vi "FGV SystemEinstellungenV2.vi"(6 "Aktion":T7, 8 "error in (no error)":errorcluster caption="Fehler (Eingang, kein Fehler)", 10 "Gasteiler definition":T1 {"Gasteiler Letzte Wartung" format="%<%x %.3X>T"}, 11 "AnalysatorDefinition":T3) -> (0 "error out":errorcluster caption="Fehler (Ausgang)", 2 "Gasteiler":T2 {"GasteilerDefinitionsListe"."Gasteiler Letzte Wartung" format="%<%x %.3X>T"}, 3 "Analysatoren":T5, 4 "Untertitel":T6, 5 "Index Neuer analysator":i32, 7 "Index Neuer Gasteiler":i32)   [LabVIEW 2020, in "System Einstellungen V2.lvlib"]
uses:
  System Einstellungen V2.lvlib
  Aktion FGV SystemEinstellungenV2.ctl
  AnalysatorDefinition.ctl
  Gasteiler.ctl
  <vilib>/Utility/miscctls.llb/LVComboBoxStrsAndValuesArrayTypeDef.ctl
  EPA 1065/Allgemeine VIs/Aktion Wertaenderung Gasliste.ctl
  Aktioen FGV System.ctl
  SysLog/SysLog Interface.ctl
  Allgemein/allgemeine Sub-VIs.lvlib
  SysLog/SysLog.lvlib
  EPA 1065/EPA 1065.lvlib
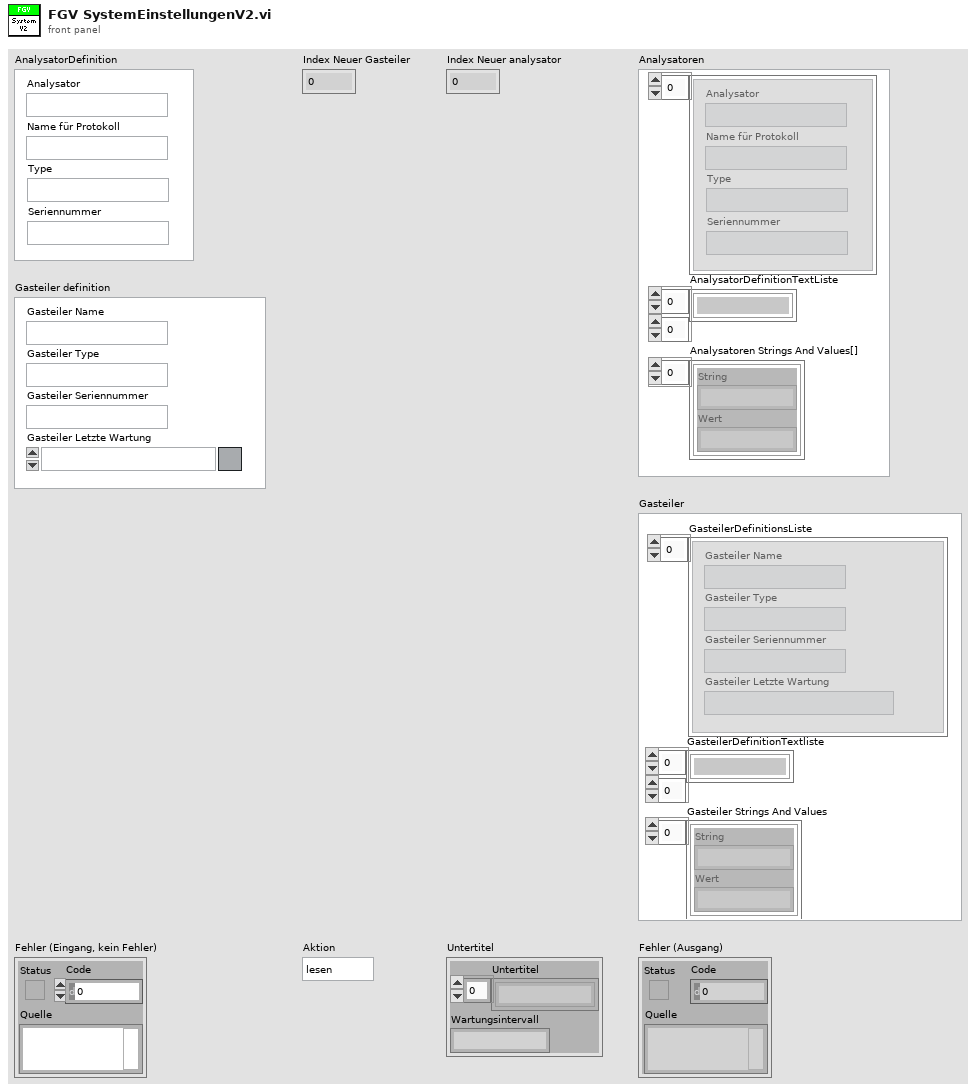
[diagram p1: front panel]
types:
  T1 = typedef "System Einstellungen V2.lvlib/Gasteiler.ctl" = cluster{"Gasteiler Name":string, "Gasteiler Type":string, "Gasteiler Seriennummer":string, "Gasteiler Letzte Wartung":timestamp}
  T2 = cluster{"GasteilerDefinitionsListe":T1[], "GasteilerDefinitionTextliste":string[][], "Gasteiler Strings And Values":cluster{"String":string, "Wert":string}[]}
  T3 = typedef "System Einstellungen V2.lvlib/AnalysatorDefinition.ctl" = cluster{"Analysator":string, "Name für Protokoll":string, "Type":string, "Seriennummer":string}
  T4 = typedef "LVComboBoxStrsAndValuesArrayTypeDef.ctl" = cluster{"String":string, "Value":string}[]
  T5 = cluster{"AnalysatorDefinitionListe":T3[], "AnalysatorDefinitionTextListe":string[][], "Analysatoren Strings And Values[]":T4}
  T6 = cluster{"Untertitel":string[], "Wartungsintervall":string}
  T7 = typedef "System Einstellungen V2.lvlib/Aktion FGV SystemEinstellungenV2.ctl" = enum16{"lesen", "Analysatoren schreiben", "Analysator ändern", "Analysatoren löschen", "laden", "speichern", "Untertitel", "Analysatoren", "Neue Analysatoren", "Gasteiler schreiben", "Gasteiler ändern", "Gasteiler löschen", "Gasteiler", "Gasteiler exportieren", "Gasteiler importieren"}
  T8 = enum16{"open", "replace", "create", "open or create", "replace or create", "replace or create with confirmation"}
  T9 = typedef "EPA 1065.lvlib/Aktion Wertaenderung Gasliste.ctl" = enum16{"Init", "lesen", "Gasliste geändert", "ARN inaktiv", "LEAK inaktiv", "Interference 366 inaktiv", "T90 inaktiv", "Interference 375 inaktiv", "Chiller inaktiv", "FID O2 inaktiv", "FID Opti inaktiv", "Drift inaktiv", "Pre Test inaktiv", "LinV2 inaktiv"}
  T10 = typedef "System Einstellungen V2.lvlib/Aktioen FGV System.ctl" = enum16{"lesen", "laden", "speichern", "Optionen schreiben", "Zeitstempel", "Reset BMP", "Reset SQP", "Wartung", "Werkseinstellung"}
  T11 = typedef "SysLog.lvlib/SysLog Interface.ctl" = cluster{"FehlermeldungsCode":i32, "ErfolgsmeldungsCode":i32, "ParameterListenString":string, "Anzeige":bool, "SysLogIcon":enum16{"OK", "Warnung", "Fehler"}, "intern":bool}
  T12 = cluster{"Gasteiler Name":string, "Gasteiler Name":string}
  T13 = cluster{"Analysator":string, "Analysator":string}[]
  T14 = typedef "System Einstellungen V2.lvlib/Optionen.ctl" = cluster{"Störmeldep.":bool, "Betriebszustände":bool, "AK in ppm":bool, "log Cal-Gas":bool, "log 0-Gas":bool, "Durchflusssensor 0-5V":bool, "PNS?":bool, "Mit N2 spülen":bool, "TRE08":bool, "Amium 10-Fach":bool, "Verticale Scrollbar aktiv":bool, "Loggingtakt":bool, "AK Rezeptwechsel gleich wie MKS":bool, "NG ECO":bool}
  T15 = cluster{"Cluster Array (Ausgang)":T1[], "Gasteiler definition":string[][], cluster{"Gasteiler Name":string, "Gasteiler Name":string}[]}
  T16 = cluster{"AnalysatorDefinition Array out":T3[], "Analysator String Array out":string[][], "Analysatoren Strings And Values[]":cluster{"Analysator":string, "Analysator":string}[]}
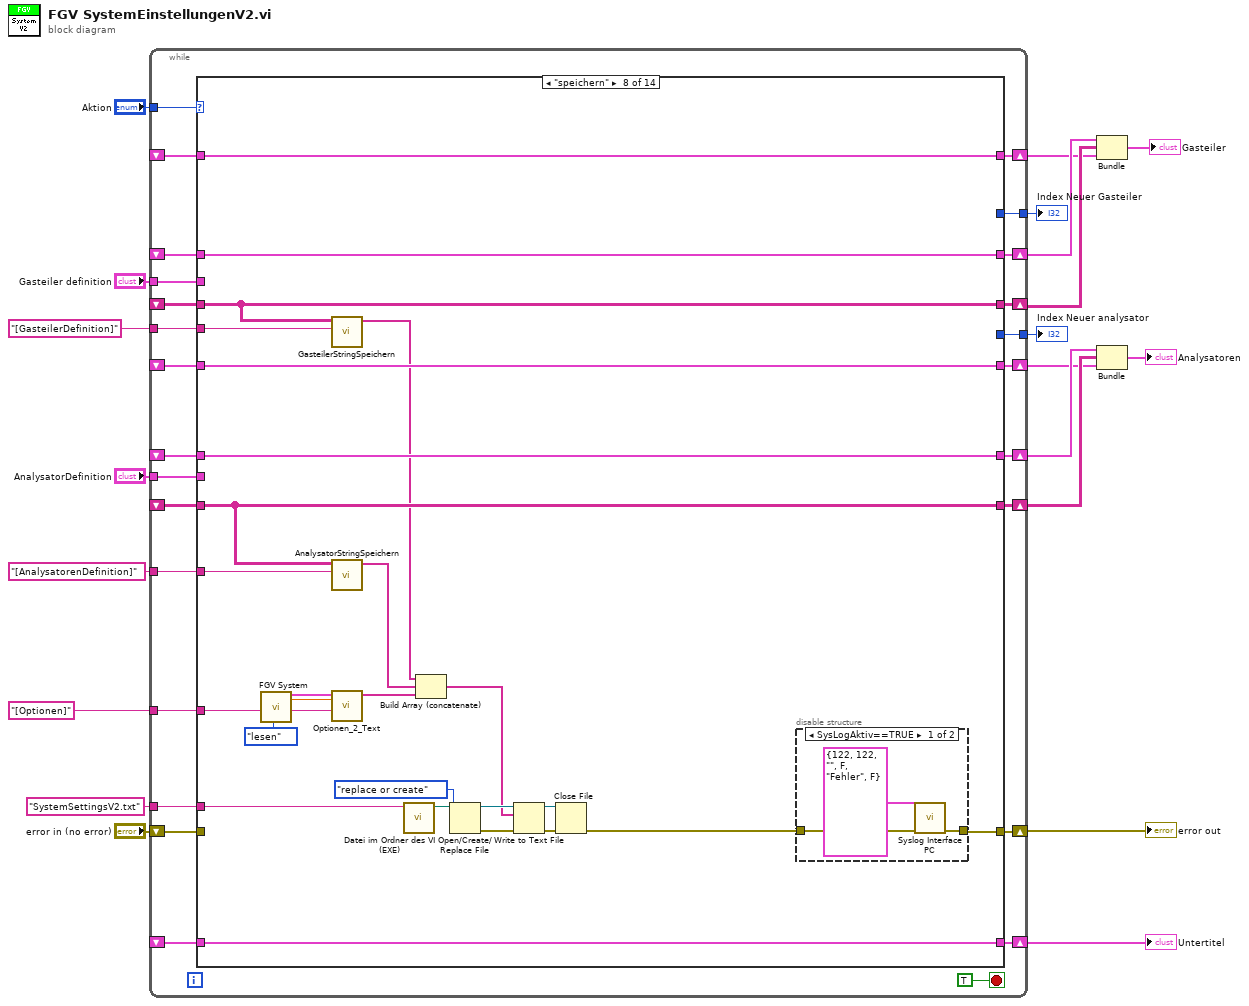
[diagram p0: block diagram]
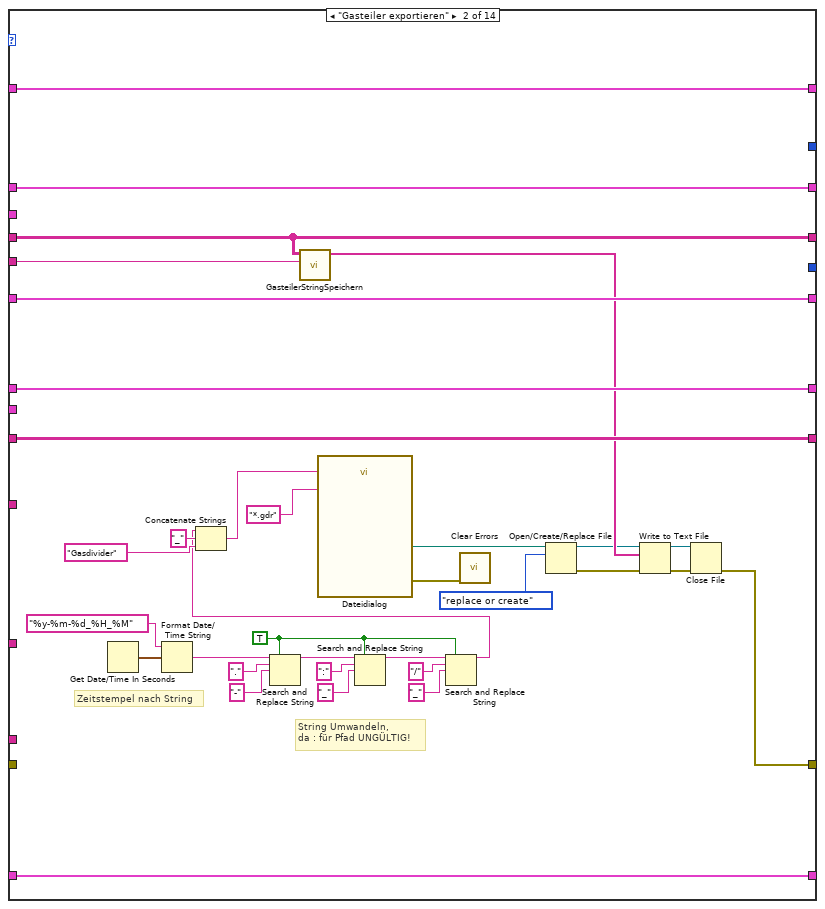
[diagram p3: hidden frame]
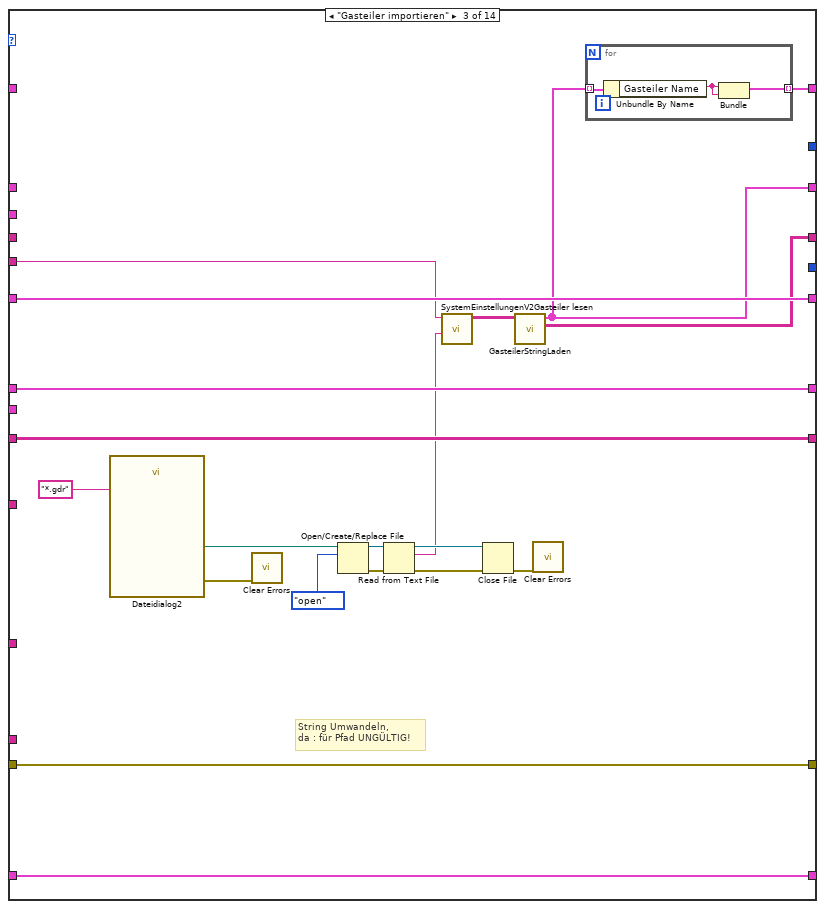
[diagram p4: hidden frame]
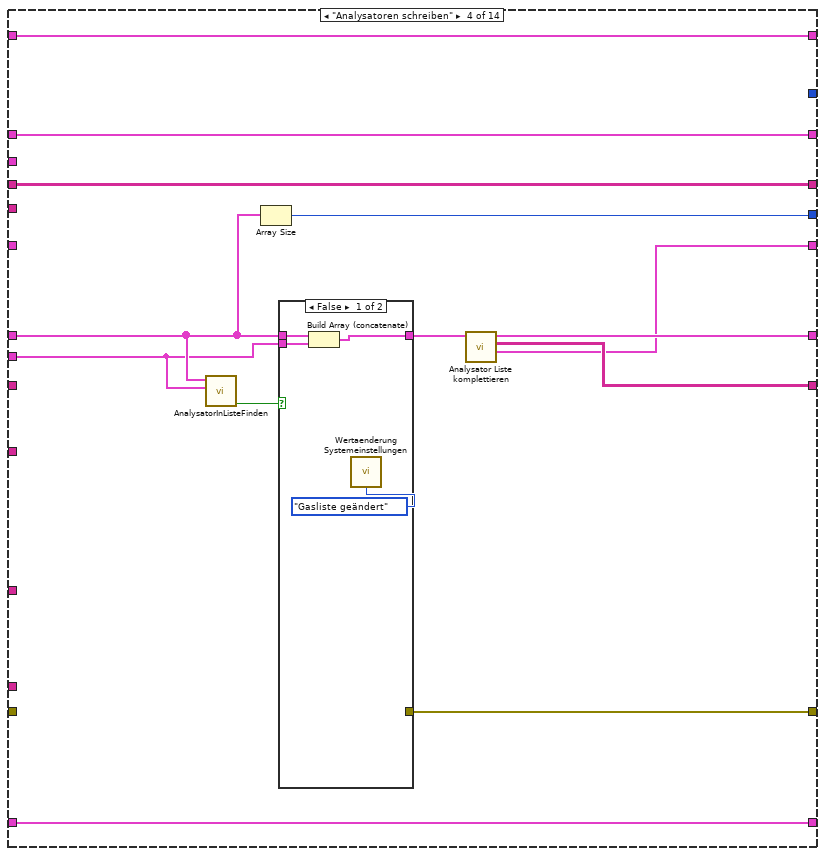
[diagram p5: hidden frame]
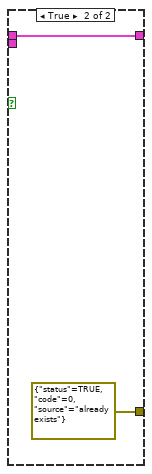
[diagram p6: hidden frame]
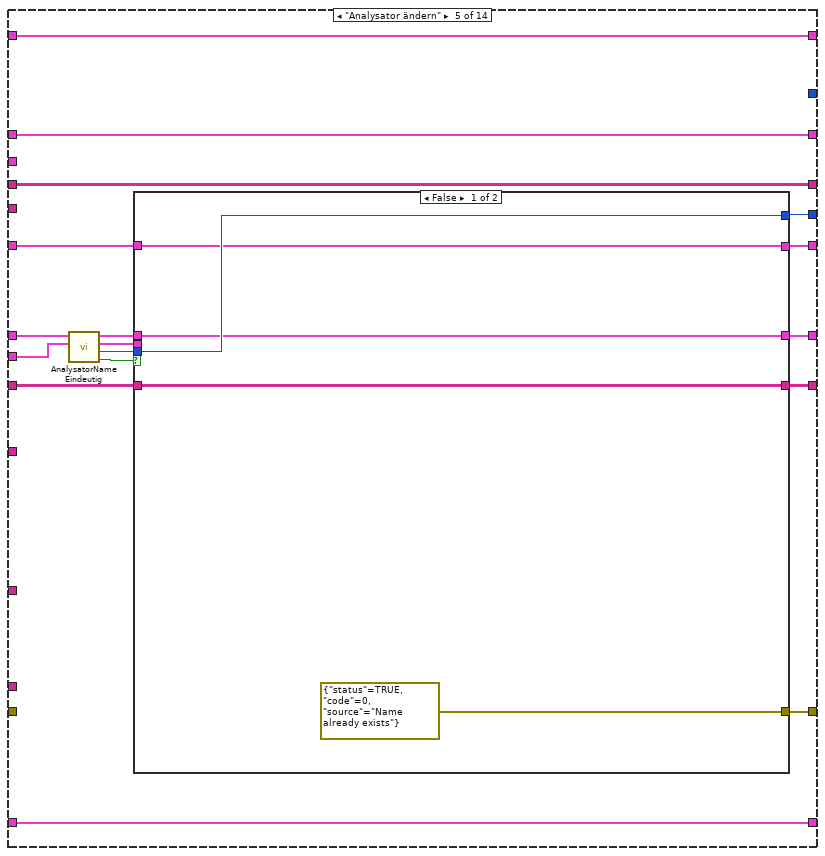
[diagram p7: hidden frame]
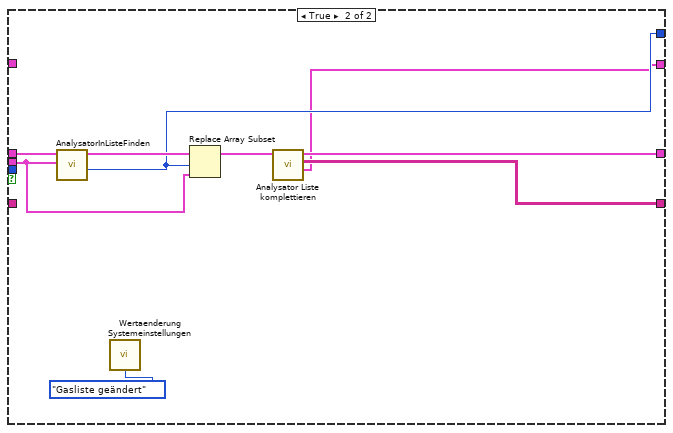
[diagram p8: hidden frame]
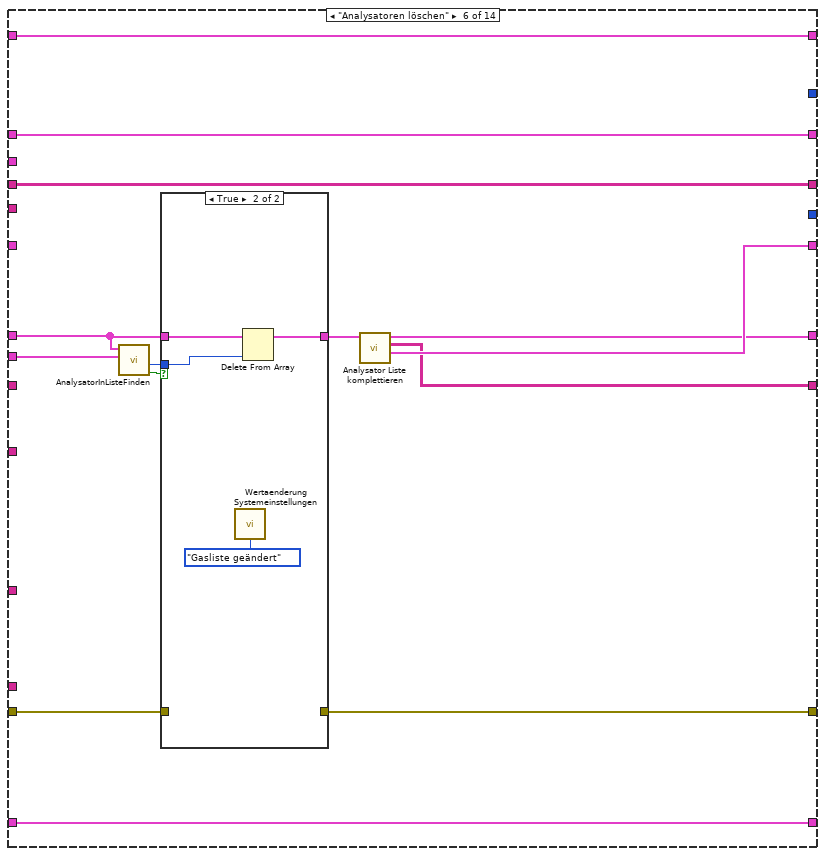
[diagram p9: hidden frame]
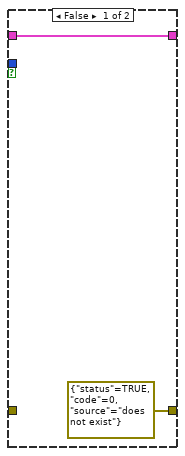
[diagram p10: hidden frame]
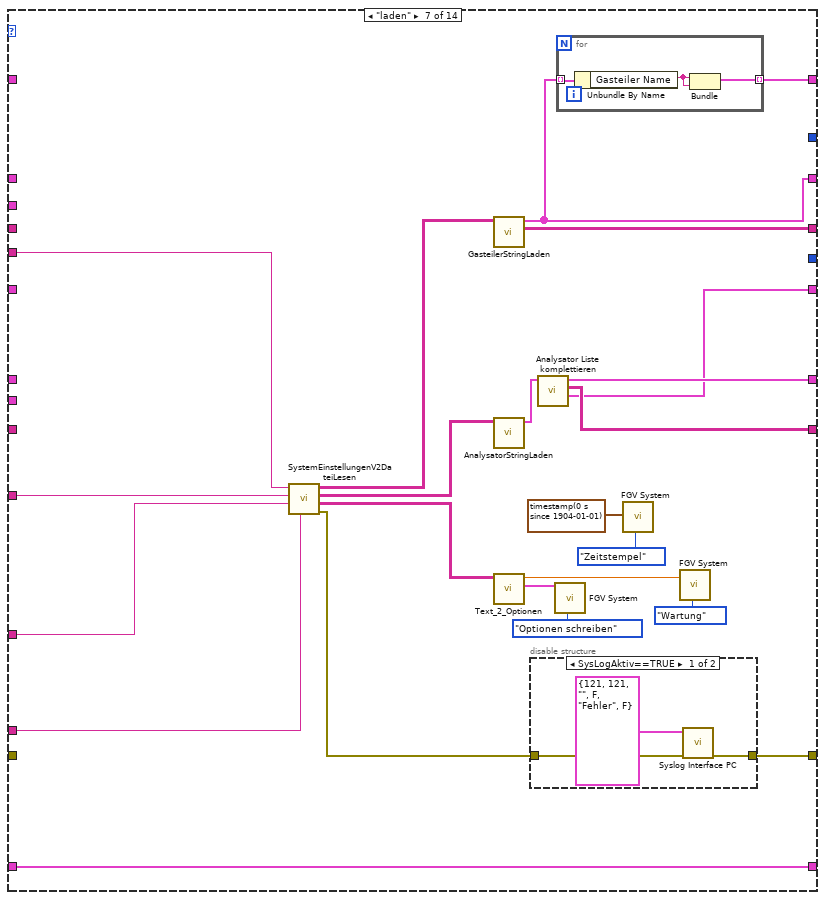
[diagram p11: hidden frame]
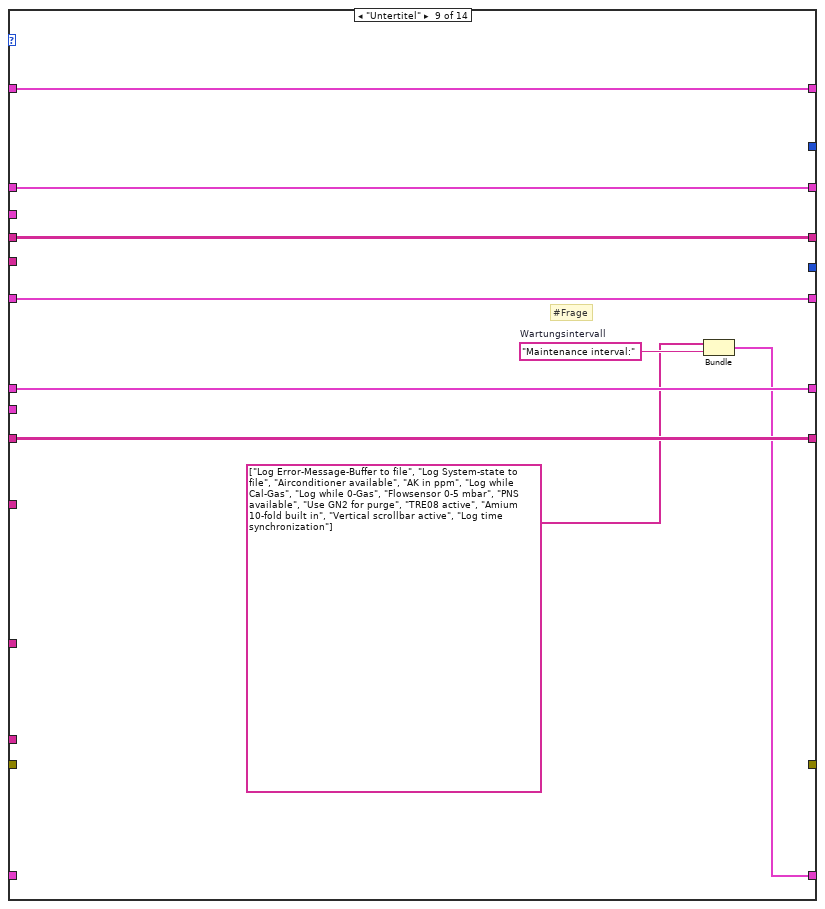
[diagram p14: hidden frame]
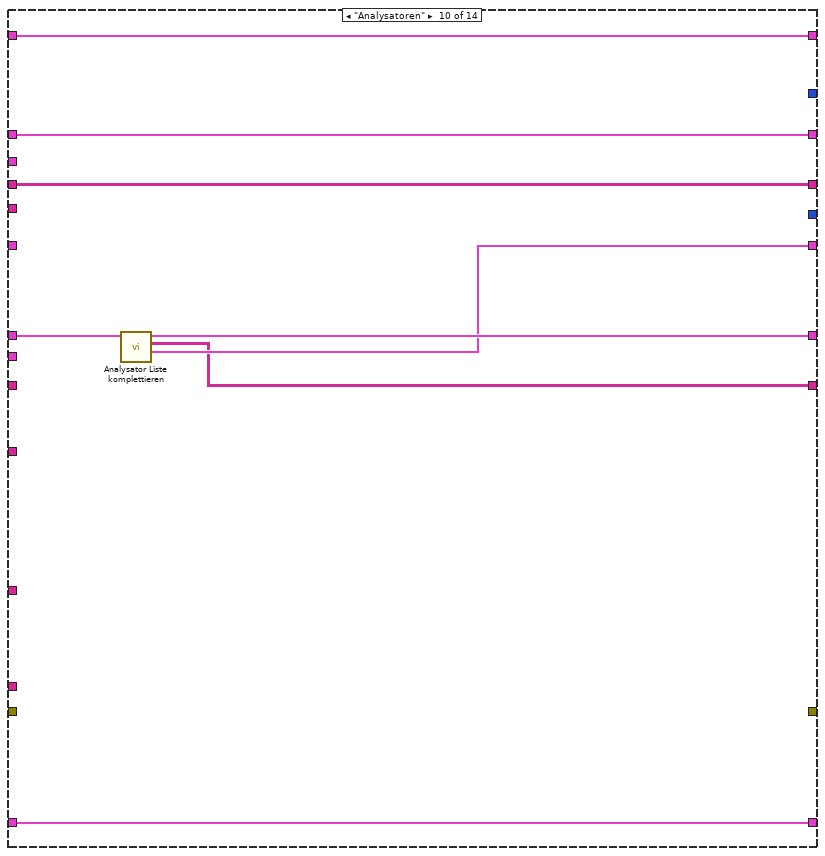
[diagram p15: hidden frame]
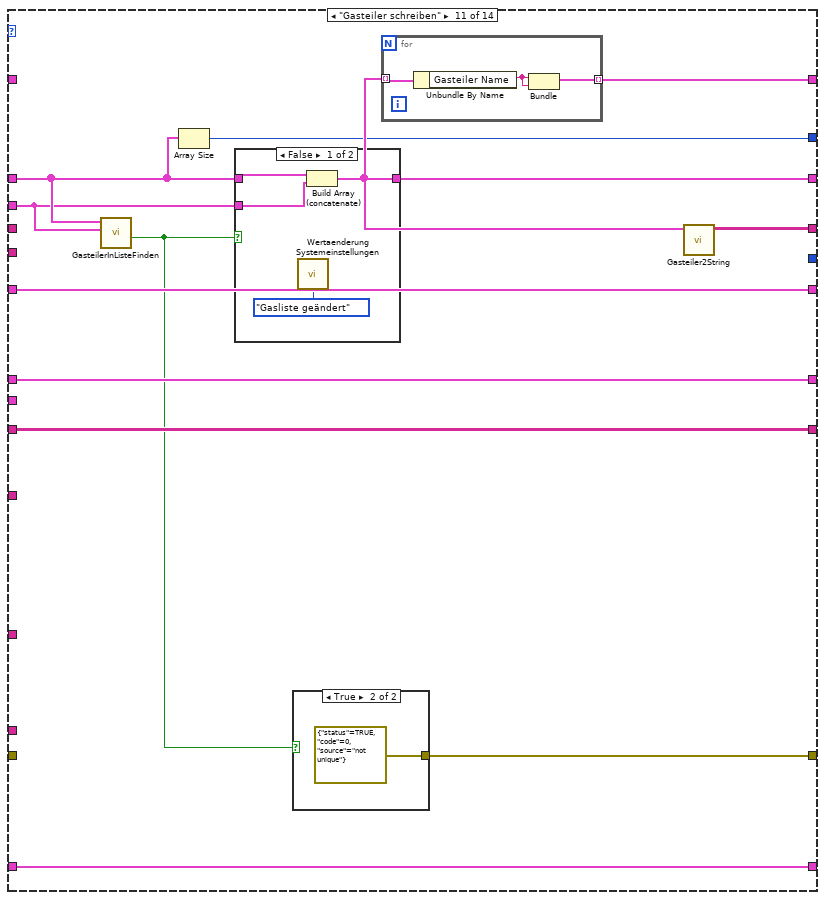
[diagram p16: hidden frame]
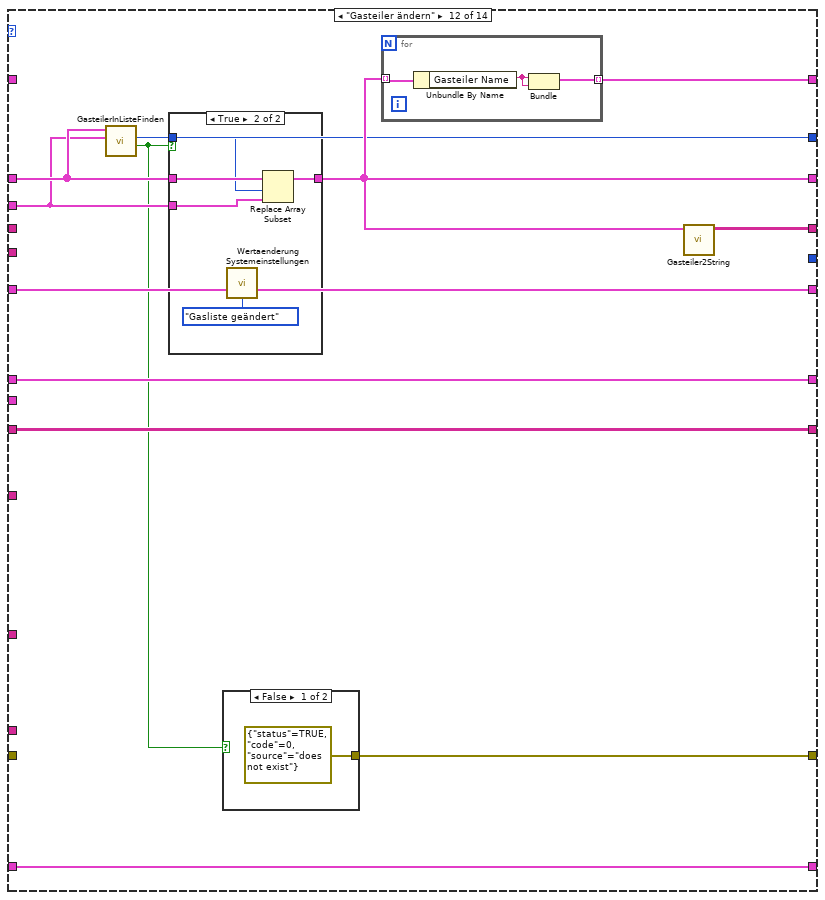
[diagram p19: hidden frame]
diagram:
  n1 = while {
    tunnel: "Aktion" -> [w45]
    shift-right: [w44] -> w12
    shift-left: _ -> [w43]
    shift-right: [w42] -> w11
    shift-left: _ -> [w41]
    shift-right: [w39] -> w18
    shift-left: "error in (no error)" -> [w40]
    tunnel: "SystemSettingsV2.txt" ("Dateiname") -> [w38]
    tunnel: "[AnalysatorenDefinition]" -> [w37]
    tunnel: "AnalysatorDefinition" -> [w36]
    tunnel: "[Optionen]" -> [w35]
    shift-right: [w34] -> w13
    shift-left: _ -> [w33]
    shift-right: [w32] -> w10
    shift-left: _ -> [w31]
    tunnel: "Gasteiler definition" -> [w30]
    shift-right: [w29] -> w7
    shift-left: _ -> [w28]
    shift-right: [w27] -> w6
    shift-left: _ -> [w26]
    shift-right: [w25] -> w5
    shift-left: _ -> [w24]
    tunnel: "[GasteilerDefinition]" -> [w23]
    tunnel: [w22] -> w2
    tunnel: [w21] -> w1
    stop <- TRUE stop-if-true
    n2 = case shown="\"speichern\"" w45 {
      tunnel: [w54 w88 w108 w114 w137 w163 w184 w237 w250 w253 w270 w291 w314 w330] -> w44
      tunnel: w43 -> [w54 w88 w108 w119 w142 w173 _ w237 w250 w254 w270 w291 w314 w330]
      tunnel: [w53 w87 w107 w113 w135 w162 w183 w229 w249 w251 w269 w290 w313 w329] -> w42
      tunnel: w41 -> [w53 w87 w107 _ w131 _ _ w229 w249 _ w269 w290 w313 w329]
      tunnel: w40 -> [w52 _ w106 _ _ w175 _ _ _ _ _ _ w306 _]
      tunnel: [w52 w55 w106 w116 w146 w174 w186 w214 _ _ w259 w287 w307 _] -> w39
      tunnel: w38 -> [_ _ _ _ _ _ w204 w230 _ _ _ _ _ _]
      tunnel: w37 -> [_ _ _ _ _ _ w190 w212 _ _ _ _ _ _]
      tunnel: w36 -> [_ _ _ w118 w141 w172 _ _ _ _ _ _ _ _]
      tunnel: w35 -> [_ _ _ _ _ _ w189 w222 _ _ _ _ _ _]
      tunnel: [w51 w86 w105 w124 w147 w171 w196 w221 w248 w258 w268 w289 w312 w328] -> w34
      tunnel: w33 -> [w51 w86 w105 w124 w147 w171 w196 w221 _ w258 w268 w289 w312 w328]
      tunnel: [w50 w85 w104 w112 w134 w165 w182 w220 w246 w252 w267 w288 w311 w327] -> w32
      tunnel: w31 -> [w50 w85 w104 _ w132 _ _ w220 w246 _ w267 w288 w311 w327]
      tunnel: w30 -> [_ _ _ _ _ _ _ _ _ _ w262 w282 w308 _]
      tunnel: [w49 w63 w92 w123 w145 w170 w192 w219 w245 w257 w266 w286 w302 w325] -> w29
      tunnel: w28 -> [w49 w63 _ w123 w145 w170 _ w219 w245 w257 w263 w283 w305 w325]
      tunnel: [w48 w62 w91 w122 w144 w169 w193 w217 w244 w256 w265 w285 w303 w326] -> w27
      tunnel: w26 -> [w48 w62 _ w122 w144 w169 _ w217 w244 w256 _ _ _ w326]
      tunnel: [w47 w64 w93 w121 w143 w168 w191 w218 w243 w255 w264 w284 w304 w324] -> w25
      tunnel: w24 -> [w47 w64 _ w121 w143 w168 _ w218 w243 w255 _ _ _ _]
      tunnel: w23 -> [_ w61 w90 _ _ _ w195 w213 _ _ _ _ _ _]
      tunnel: [_ _ _ _ _ _ _ _ _ _ w261 w281 _ _] -> w22
      tunnel: [_ _ _ w120 w136 _ _ _ _ _ _ _ _ _] -> w21
      frame "lesen", Default {
      }
      frame "Gasteiler exportieren" {
        w72 = TRUE ("Alle ersetzen? (F)")
        # "String Umwandeln, \nda : für Pfad UNGÜLTIG!"
        # "Zeitstempel nach String"
        n3 = Get Date/Time In Seconds() -> (seconds since 1Jan1904=w82:timestamp)
        n4 = Format Date/Time String(time format string (%c)="%y-%m-%d_%H_%M" ("Zeitformatierungs-String (%c)"), seconds (now)=w82) -> (date/time string=w81:string)  [unwired: 1 in]
        n5 = Search and Replace String(replace all?=w72, input string=w81, search string="." ("Such-String"), replace string="-" ("String ersetzen(\"\")")) -> (result string=w78:string)  [unwired: 4 in, 3 out]
        n6 = call "GasteilerStringSpeichern.vi"("Abschnitt"=w61, "GasteilerDefinition"=w62) -> ("Gasdivider Text to save"=w60:string[])  [unwired: 9 in]
        n7 = Search and Replace String(replace all?=w72, input string=w78, search string=":" ("Such-String"), replace string="_" ("String ersetzen(\"\")")) -> (result string=w73:string)  [unwired: 4 in, 3 out]
        n8 = Search and Replace String(replace all?=w72, input string=w73, search string="/" ("Such-String"), replace string="_" ("String ersetzen(\"\")")) -> (result string=w68:string)  [unwired: 4 in, 3 out]
        n9 = Concatenate Strings(w68, "_" ("String"), "Gasdivider" ("default name")) -> (w67:string)
        n10 = call "Dateidialog"("default name"=w67, "pattern (all files)"="*.gdr") -> ("selected path"=w66:path, "error out"=w83:errorcluster)  [unwired: 10 in, 2 out]
        n11 = call <vilib>:"Clear Errors.vi"("error in (no error)"=w83) -> ()  [unwired: 5 in, 2 out]
        n12 = Open/Create/Replace File(file path (use dialog)=w66, operation (0:open)=T8."replace or create" ("Operation (0:open)")) -> (refnum out=w59:refnum<file>, error out=w58:errorcluster)  [unwired: 4 in, 1 out]
        n13 = Write to Text File(file (use dialog)=w59, text=w60, error in=w58) -> (refnum out=w56:refnum<file>, error out=w57:errorcluster)  [unwired: 1 in, 1 out]
        n14 = Close File(refnum=w56, error in=w57) -> (error out=w55:errorcluster)  [unwired: 1 out]
      }
      frame "Gasteiler importieren" {
        # "String Umwandeln, \nda : für Pfad UNGÜLTIG!"
        n15 = call "Dateidialog2"("pattern (all files)"="*.gdr") -> ("selected path"=w101:path, "error out"=w102:errorcluster)  [unwired: 11 in, 2 out]
        n16 = call <vilib>:"Clear Errors.vi"("error in (no error)"=w102) -> ()  [unwired: 5 in, 2 out]
        n17 = Open/Create/Replace File(file path (use dialog)=w101, operation (0:open)=T8."open" ("Operation (0:open)")) -> (refnum out=w98:refnum<file>, error out=w97:errorcluster)  [unwired: 4 in, 1 out]
        n18 = Read from Text File(file (use dialog)=w98, error in=w97) -> (refnum out=w95:refnum<file>, text=w89:string, error out=w96:errorcluster)  [unwired: 2 in, 1 out]
        n19 = call "SystemEinstellungenV2Gasteiler lesen.vi"("Tabellen-String"=w89, "[GasteilerDefinition]"=w90) -> ("[GasteilerDefinition]"=w94:string[][])  [unwired: 8 in, 1 out]
        n20 = Close File(refnum=w95, error in=w96) -> (error out=w99:errorcluster)  [unwired: 1 out]
        n21 = call "GasteilerStringLaden.vi"("Array (Eingang)"=w94) -> ("string array"=w91:string[][], "Cluster Array (Ausgang)"=w92:T1[])  [unwired: 9 in]
        n22 = call <vilib>:"Clear Errors.vi"("error in (no error)"=w99) -> ()  [unwired: 5 in, 2 out]
        n23 = for {
          tunnel: w92 -> [w111] mode=indexing
          tunnel: [w110] -> w93 mode=indexing
          n24 = Unbundle By Name(w111) -> ("Gasteiler Name"=w109:string)
          n25 = Bundle("Gasteiler Name"=w109, "Gasteiler Name"=w109) -> (w110:T12)  [unwired: 1 in]
        }
      }
      frame "Analysatoren schreiben" {
        n26 = call "AnalysatorInListeFinden.vi"("AnalysatorDefinition"=w118, "AnalysatorListe"=w119) -> ("gefunden"=w117:bool)  [unwired: 6 in, 3 out]
        n27 = Array Size(array=w119) -> (size(s)=w120:i32)
        n28 = case shown="False" w117 {
          tunnel: [w128 w130] -> w115
          tunnel: w119 -> [w127 w130]
          tunnel: w118 -> [w126 _]
          tunnel: [_ errorcluster {"status"=TRUE, "code"=0, "source"="already exists"} ("error in (no error)")] -> w116
          frame False {
            n29 = Build Array (concatenate)(w127, w126) -> (w128:T3[])
            n30 = call "Wertaenderung Systemeinstellungen.vi"("Aktion"=Aktion_Wertaenderung_Gasliste."Gasliste geändert") -> ()  [unwired: 13 in, 2 out]
          }
          frame True {
          }
        }
        n31 = call "Analysator Liste komplettieren.vi"("AnalysatorDefinition Array in"=w115) -> ("Analysatoren Strings And Values[]"=w112:T13, "Analysator String Array out"=w113:string[][], "AnalysatorDefinition Array out"=w114:T3[])  [unwired: 8 in]
      }
      frame "Analysator ändern" {
        n32 = call "AnalysatorNameEindeutig.vi"("AnalysatorDefinition"=w141, "AnalysatorListe"=w142) -> ("unique"=w140:bool, "Index"=w133:i32, "AnalysatorDefinition out"=w139:T3, "AnalysatorListe out"=w138:T3[])  [unwired: 6 in]
        n33 = case shown="False" w140 {
          tunnel: [errorcluster {"status"=TRUE, "code"=0, "source"="Name already exists"} ("error in (no error)") _] -> w146
          tunnel: w139 -> [_ w153]
          tunnel: w138 -> [w148 w159]
          tunnel: [w148 w156] -> w137
          tunnel: [w152 w158] -> w136
          tunnel: [w149 w155] -> w135
          tunnel: [w150 w154] -> w134
          tunnel: w133 -> [w152 _]
          tunnel: w132 -> [w150 _]
          tunnel: w131 -> [w149 _]
          frame False {
          }
          frame True {
            n34 = call "AnalysatorInListeFinden.vi"("AnalysatorDefinition"=w153, "AnalysatorListe"=w159) -> ("Index"=w158:i32, "AnalysatorListe out"=w160:T3[])  [unwired: 6 in, 2 out]
            n35 = call "Wertaenderung Systemeinstellungen.vi"("Aktion"=Aktion_Wertaenderung_Gasliste."Gasliste geändert") -> ()  [unwired: 13 in, 2 out]
            n36 = Replace Array Subset(array=w160, new element=w153, index=w158) -> (w157:T3[])
            n37 = call "Analysator Liste komplettieren.vi"("AnalysatorDefinition Array in"=w157) -> ("Analysatoren Strings And Values[]"=w154:T13, "Analysator String Array out"=w155:string[][], "AnalysatorDefinition Array out"=w156:T3[])  [unwired: 8 in]
          }
        }
      }
      frame "Analysatoren löschen" {
        n38 = call "AnalysatorInListeFinden.vi"("AnalysatorDefinition"=w172, "AnalysatorListe"=w173) -> ("gefunden"=w167:bool, "Index"=w166:i32)  [unwired: 6 in, 2 out]
        n39 = case shown="True" w167 {
          tunnel: [w177 w180] -> w164
          tunnel: w173 -> [w177 w181]
          tunnel: [errorcluster {"status"=TRUE, "code"=0, "source"="does not exist"} ("error in (no error)") _] -> w174
          tunnel: w175 -> [_ _]
          tunnel: w166 -> [_ w178]
          frame False {
          }
          frame True {
            n40 = call "Wertaenderung Systemeinstellungen.vi"("Aktion"=Aktion_Wertaenderung_Gasliste."Gasliste geändert") -> ()  [unwired: 13 in, 2 out]
            n41 = Delete From Array(array=w181, index=w178) -> (array with subset deleted=w180:T3[])  [unwired: 1 in, 1 out]
          }
        }
        n42 = call "Analysator Liste komplettieren.vi"("AnalysatorDefinition Array in"=w164) -> ("Analysatoren Strings And Values[]"=w165:T13, "Analysator String Array out"=w162:string[][], "AnalysatorDefinition Array out"=w163:T3[])  [unwired: 8 in]
      }
      frame "laden" {
        n43 = call "SystemEinstellungenV2DateiLesen.vi"("Dateiname"=w204, "[Optionen]"=w189, "[AnalysatorenDefinition]"=w190, "[GasteilerDefinition]"=w195) -> ("Fehler (Ausgang)"=w203:errorcluster, "[Optionen]"=w187:string[][], "[AnalysatorenDefinition]"=w188:string[][], "[GasteilerDefinition]"=w194:string[][])  [unwired: 4 in]
        n44 = call "GasteilerStringLaden.vi"("Array (Eingang)"=w194) -> ("string array"=w193:string[][], "Cluster Array (Ausgang)"=w192:T1[])  [unwired: 9 in]
        n45 = call "AnalysatorStringLaden.vi"("Array (Eingang)"=w188) -> ("Cluster Array (Ausgang)"=w185:T3[])  [unwired: 9 in, 1 out]
        n46 = call "Text_2_Optionen.vi"("Optionen String"=w187) -> ("Optionen"=w197:T14, "Wartungsintervall:"=w198:sgl)  [unwired: 8 in, 1 out]
        n47 = disable-structure shown="SysLogAktiv==TRUE" {
          disable-tunnel: w203 -> [w210 w211]
          disable-tunnel: [w208 w211] -> w186
          frame condition #0 (active) {
            n48 = call "Syslog Interface PC.vi"("Fehler (in)"=w210, "Cluster (in)"=T11 {"FehlermeldungsCode"=121, "ErfolgsmeldungsCode"=121, "ParameterListenString"="", "Anzeige"=FALSE, "SysLogIcon"=enum."Fehler", "intern"=FALSE}) -> ("Fehler (out)"=w208:errorcluster)  [unwired: 9 in]
          }
          frame condition #1 {
          }
        }
        n49 = call "Analysator Liste komplettieren.vi"("AnalysatorDefinition Array in"=w185) -> ("Analysatoren Strings And Values[]"=w182:T13, "Analysator String Array out"=w183:string[][], "AnalysatorDefinition Array out"=w184:T3[])  [unwired: 8 in]
        n50 = call "FGV System.vi"("Optionen"=w197, "Aktionen"=Aktioen_FGV_System."Optionen schreiben") -> ()  [unwired: 11 in, 7 out]
        n51 = for {
          tunnel: w192 -> [w207] mode=indexing
          tunnel: [w206] -> w191 mode=indexing
          n52 = Unbundle By Name(w207) -> ("Gasteiler Name"=w205:string)
          n53 = Bundle("Gasteiler Name"=w205, "Gasteiler Name"=w205) -> (w206:T12)  [unwired: 1 in]
        }
        n54 = call "FGV System.vi"("Zeitstempel"=timestamp(0 s since 1904-01-01), "Aktionen"=Aktioen_FGV_System."Zeitstempel") -> ()  [unwired: 11 in, 7 out]
        n55 = call "FGV System.vi"("Wartungsintervall:"=w198, "Aktionen"=Aktioen_FGV_System."Wartung") -> ()  [unwired: 11 in, 7 out]
      }
      frame "speichern" {
        n56 = call "FGV System.vi"("Aktionen"=Aktioen_FGV_System."lesen") -> ("Optionen"=w224:T14, "Wartungsintervall:"=w223:sgl)  [unwired: 12 in, 5 out]
        n57 = call "GasteilerStringSpeichern.vi"("Abschnitt"=w213, "GasteilerDefinition"=w217) -> ("Gasdivider Text to save"=w216:string[])  [unwired: 9 in]
        n58 = call "AnalysatorStringSpeichern.vi"("Abschnitt"=w212, "AnalysatorDefinition"=w229) -> ("Analyser Text to save"=w228:string[])  [unwired: 9 in]
        n59 = call "Optionen_2_Text.vi"("Abschnitt"=w222, "Wartungsintervall:"=w223, "Optionen"=w224) -> ("Array"=w215:string[])  [unwired: 7 in, 1 out]
        n60 = call "Datei im Ordner des VI (EXE).vi"("Dateiname"=w230) -> ("Dateipfad im Ordner des Haupt-VIs"=w236:path)  [unwired: 8 in, 2 out]
        n61 = Build Array (concatenate)(w216, w228, w215) -> (w227:string[])
        n62 = Open/Create/Replace File(file path (use dialog)=w236, operation (0:open)=T8."replace or create" ("Operation (0:open)")) -> (refnum out=w235:refnum<file>, error out=w234:errorcluster)  [unwired: 4 in, 1 out]
        n63 = Write to Text File(file (use dialog)=w235, text=w227, error in=w234) -> (refnum out=w232:refnum<file>, error out=w233:errorcluster)  [unwired: 1 in, 1 out]
        n64 = Close File(refnum=w232, error in=w233) -> (error out=w225:errorcluster)  [unwired: 1 out]
        n65 = disable-structure shown="SysLogAktiv==TRUE" {
          disable-tunnel: w225 -> [w240 w241]
          disable-tunnel: [w238 w241] -> w214
          frame condition #0 (active) {
            n66 = call "Syslog Interface PC.vi"("Fehler (in)"=w240, "Cluster (in)"=T11 {"FehlermeldungsCode"=122, "ErfolgsmeldungsCode"=122, "ParameterListenString"="", "Anzeige"=FALSE, "SysLogIcon"=enum."Fehler", "intern"=FALSE}) -> ("Fehler (out)"=w238:errorcluster)  [unwired: 9 in]
          }
          frame condition #1 {
          }
        }
      }
      frame "Untertitel" {
        w247 = "Maintenance interval:"  # Wartungsintervall
        # "#Frage"
        n67 = Bundle(string[] ["Log Error-Message-Buffer to file", "Log System-state to file", "Airconditioner available", "AK in ppm", "Log while Cal-Gas", "Log while 0-Gas", "Flowsensor 0-5 mbar", "PNS available", "Use GN2 for purge", "TRE08 active", "Amium 10-fold built in", "Vertical scrollbar active", "Log time synchronization"], "Wartungsintervall"=w247) -> (w248:cluster{string[], "Wartungsintervall":string})  [unwired: 1 in]
      }
      frame "Analysatoren" {
        n68 = call "Analysator Liste komplettieren.vi"("AnalysatorDefinition Array in"=w254) -> ("Analysatoren Strings And Values[]"=w252:T13, "Analysator String Array out"=w251:string[][], "AnalysatorDefinition Array out"=w253:T3[])  [unwired: 8 in]
      }
      frame "Gasteiler schreiben" {
        n69 = call "GasteilerInListeFinden.vi"("Gasteiler definition"=w262, "GasteilerListe"=w263) -> ("gefunden"=w260:bool)  [unwired: 7 in, 2 out]
        n70 = Array Size(array=w263) -> (size(s)=w261:i32)
        n71 = case shown="False" w260 {
          tunnel: [w275 w276] -> w266
          tunnel: w263 -> [w274 w276]
          tunnel: w262 -> [w273 _]
          frame False {
            n72 = call "Wertaenderung Systemeinstellungen.vi"("Aktion"=Aktion_Wertaenderung_Gasliste."Gasliste geändert") -> ()  [unwired: 13 in, 2 out]
            n73 = Build Array (concatenate)(w274, w273) -> (w275:T1[])
          }
          frame True {
          }
        }
        n74 = case shown="True" w260 {
          tunnel: [_ errorcluster {"status"=TRUE, "code"=0, "source"="not unique"} ("error in (no error)")] -> w259
          frame False {
          }
          frame True {
          }
        }
        n75 = for {
          tunnel: w266 -> [w279] mode=indexing
          tunnel: [w278] -> w264 mode=indexing
          n76 = Unbundle By Name(w279) -> ("Gasteiler Name"=w277:string)
          n77 = Bundle("Gasteiler Name"=w277, "Gasteiler Name"=w277) -> (w278:T12)  [unwired: 1 in]
        }
        n78 = call "Gasteiler2String.vi"("Cluster Array (Eingang)"=w266) -> ("Gasteiler definition"=w265:string[][])  [unwired: 10 in]
      }
      frame "Gasteiler ändern" {
        n79 = call "GasteilerInListeFinden.vi"("Gasteiler definition"=w282, "GasteilerListe"=w283) -> ("gefunden"=w280:bool, "Index"=w281:i32)  [unwired: 7 in, 1 out]
        n80 = case shown="True" w280 {
          tunnel: [w292 w297] -> w286
          tunnel: w283 -> [w292 w296]
          tunnel: w282 -> [_ w295]
          tunnel: w281 -> [_ w294]
          frame False {
          }
          frame True {
            n81 = call "Wertaenderung Systemeinstellungen.vi"("Aktion"=Aktion_Wertaenderung_Gasliste."Gasliste geändert") -> ()  [unwired: 13 in, 2 out]
            n82 = Replace Array Subset(array=w296, new element=w295, index=w294) -> (w297:T1[])
          }
        }
        n83 = case shown="False" w280 {
          tunnel: [errorcluster {"status"=TRUE, "code"=0, "source"="does not exist"} ("error in (no error)") _] -> w287
          frame False {
          }
          frame True {
          }
        }
        n84 = for {
          tunnel: w286 -> [w301] mode=indexing
          tunnel: [w300] -> w284 mode=indexing
          n85 = Unbundle By Name(w301) -> ("Gasteiler Name"=w299:string)
          n86 = Bundle("Gasteiler Name"=w299, "Gasteiler Name"=w299) -> (w300:T12)  [unwired: 1 in]
        }
        n87 = call "Gasteiler2String.vi"("Cluster Array (Eingang)"=w286) -> ("Gasteiler definition"=w285:string[][])  [unwired: 10 in]
      }
      frame "Gasteiler löschen" {
        n88 = call "GasteilerInListeFinden.vi"("Gasteiler definition"=w308, "GasteilerListe"=w305) -> ("gefunden"=w310:bool, "Index"=w309:i32)  [unwired: 7 in, 1 out]
        n89 = case shown="True" w310 {
          tunnel: [w319 w322] -> w302
          tunnel: w305 -> [w319 w323]
          tunnel: w309 -> [_ w321]
          tunnel: [errorcluster {"status"=TRUE, "code"=0, "source"="does not exist"} ("error in (no error)") _] -> w307
          tunnel: w306 -> [_ _]
          frame False {
          }
          frame True {
            n90 = Delete From Array(array=w323, index=w321) -> (array with subset deleted=w322:T1[])  [unwired: 1 in, 1 out]
            n91 = call "Wertaenderung Systemeinstellungen.vi"("Aktion"=Aktion_Wertaenderung_Gasliste."Gasliste geändert") -> ()  [unwired: 13 in, 2 out]
          }
        }
        n92 = for {
          tunnel: w302 -> [w317] mode=indexing
          tunnel: [w316] -> w304 mode=indexing
          n93 = Unbundle By Name(w317) -> ("Gasteiler Name"=w315:string)
          n94 = Bundle("Gasteiler Name"=w315, "Gasteiler Name"=w315) -> (w316:T12)  [unwired: 1 in]
        }
        n95 = call "Gasteiler2String.vi"("Cluster Array (Eingang)"=w302) -> ("Gasteiler definition"=w303:string[][])  [unwired: 10 in]
      }
      frame "Gasteiler" {
        n96 = for {
          tunnel: w325 -> [w333] mode=indexing
          tunnel: [w332] -> w324 mode=indexing
          n97 = Unbundle By Name(w333) -> ("Gasteiler Name"=w331:string)
          n98 = Bundle("Gasteiler Name"=w331, "Gasteiler Name"=w331) -> (w332:T12)  [unwired: 1 in]
        }
      }
    }
  }
  "error out" <- w18
  "Untertitel" <- w13
  "Index Neuer Gasteiler" <- w2
  "Index Neuer analysator" <- w1
  n99 = Bundle("Cluster Array (Ausgang)"=w7, "Gasteiler definition"=w6, w5) -> (→"Gasteiler":T15)  [unwired: 1 in]
  n100 = Bundle("AnalysatorDefinition Array out"=w12, "Analysator String Array out"=w11, "Analysatoren Strings And Values[]"=w10) -> (→"Analysatoren":T16)  [unwired: 1 in]
